vi "Calib_Ref_info.vi"(1 "Input string":string, 2 "Reference Name":string="Instrument to calibrate") -> (0 "Reference instrument":T2={"high limit (10V)"=4.0, "low limit (-10V)"=0.0, "Ch No"=4, "Off ch no"=0, "Calib filename"=path "", "Ref Instrument type"=enum."Enter Value"} {"Off ch no" min=0 max=1; "Ch No" min=0 max=7; "low limit (-10V)" min=-10 max=10 format="%.1f"; "high limit (10V)" min=-10 max=10 format="%.1f"})   [LabVIEW 2010]
uses:
  Calib_setup.ctl
  Controls/Ref_Inst_type.ctl
panel:
  in  "Ref Instrument type":T1=enum."Generic Linear"
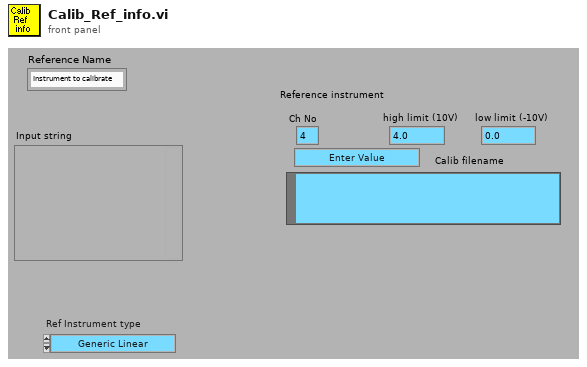
[diagram p1: front panel]
types:
  T1 = typedef "Ref_Inst_type.ctl" = enum16{"Propellor anemometer", "Pressure Transducer", "Raw voltage", "Pitot-static tube", "Preston tube", "Generic Linear", "Generic Polynomial", "Thermocouple", "LDA", "Enter Value", "ADAM Channel"}
  T2 = typedef "Calib_setup.ctl" = cluster{"high limit (10V)":sgl, "low limit (-10V)":sgl, "Ch No":i16, "Off ch no":i8, "Calib filename":path, "Ref Instrument type":T1}
  T3 = cluster{"high limit (10V)":sgl, "low limit (-10V)":sgl, "Ch No":i16, "Off ch no":i8, "Calib filename":path, "Ref Instrument type":enum16{"Propellor anemometer", "Pressure Transducer", "Raw voltage", "Pitot-static tube", "Generic Inst", "Thermocouple", "LDA", "Enter Value", "ADAM Channel"}}
  T4 = enum16{"Propellor anemometer", "Pressure Transducer", "Raw voltage", "Pitot-static tube", "Generic Inst", "Thermocouple", "LDA", "Enter Value", "ADAM Channel"}
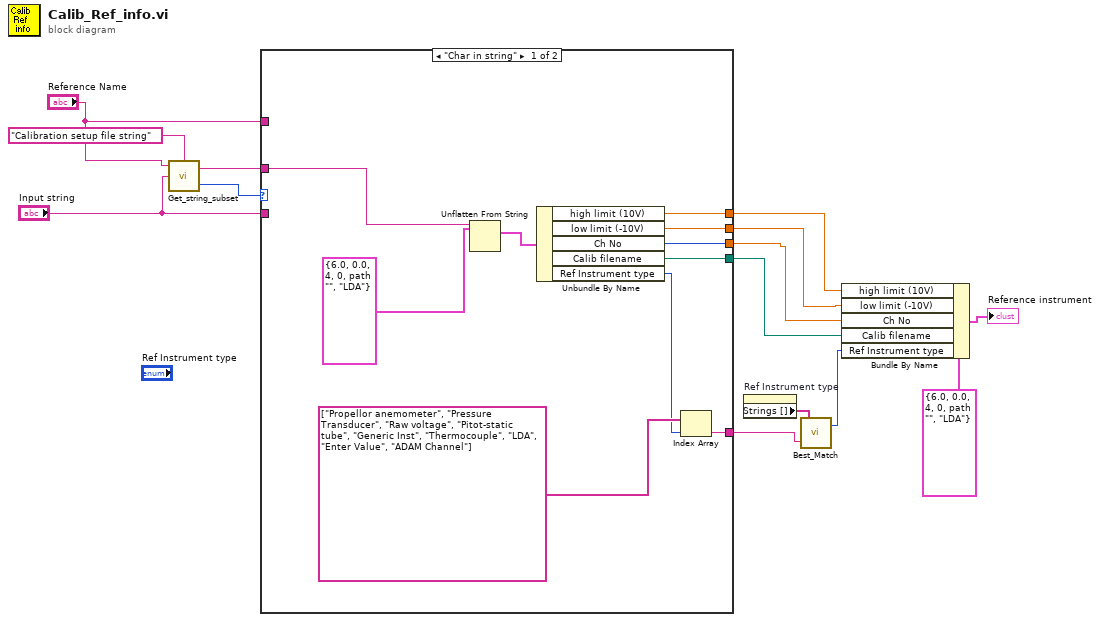
[diagram p0: block diagram]
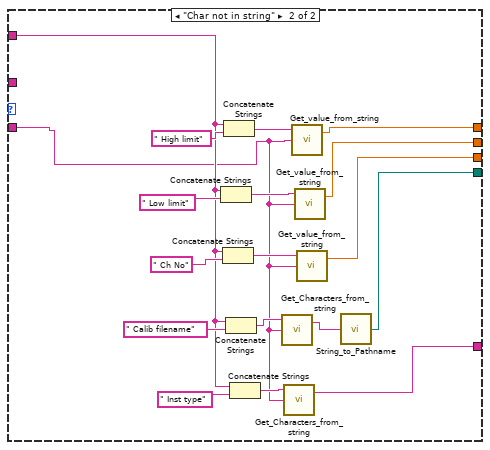
[diagram p2: hidden frame]
diagram:
  n1 = call "Get_string_subset.vi"("String Name"="Calibration setup file string", "String to split"="Input string", "File Label"="Reference Name") -> ("Status"=w13:enum16{"Char in string", "Char not in string"}, "Output string"=w12:string)  [unwired: 1 in]
  n2 = case shown="\"Char in string\"" w13 {
    tunnel: "Input string" -> [_ w30]
    tunnel: w12 -> [w24 _]
    tunnel: "Reference Name" -> [_ w34]
    tunnel: [w19 w25] -> w7
    tunnel: [w18 w26] -> w5
    tunnel: [w17 w27] -> w4
    tunnel: [w16 w28] -> w3
    tunnel: [w15 w29] -> w2
    frame "Char in string" {
      n3 = Unflatten From String(type=T3 {"high limit (10V)"=6.0, "low limit (-10V)"=0.0, "Ch No"=4, "Off ch no"=0, "Calib filename"=path "", "Ref Instrument type"=enum."LDA"} ("Ref vel for angle calib"), binary string=w24) -> (value=w22:T3)  [unwired: 1 in, 4 out]
      n4 = Unbundle By Name(w22) -> ("high limit (10V)"=w15:sgl, "low limit (-10V)"=w16:sgl, "Ch No"=w17:i16, "Calib filename"=w18:path, "Ref Instrument type"=w20:T4)
      n5 = Index Array(array=string[] ["Propellor anemometer", "Pressure Transducer", "Raw voltage", "Pitot-static tube", "Generic Inst", "Thermocouple", "LDA", "Enter Value", "ADAM Channel"] ("Strings []"), index=w20) -> (element=w19:string)
    }
    frame "Char not in string" {
      n6 = Concatenate Strings(w34, " Low limit") -> (w37:string)
      n7 = Concatenate Strings(w34, " Ch No") -> (w38:string)
      n8 = Concatenate Strings(w34, " High limit") -> (w39:string)
      n9 = Concatenate Strings(w34, " Calib filename") -> (w33:string)
      n10 = Concatenate Strings(w34, " Inst type") -> (w31:string)
      n11 = call "Get_Characters_from_string.vi"("Input string"=w30, "Variable name"=w33) -> ("Value"=w32:string)  [unwired: 1 in, 1 out]
      n12 = call "Get_Characters_from_string.vi"("Input string"=w30, "Variable name"=w31) -> ("Value"=w25:string)  [unwired: 1 in, 1 out]
      n13 = call "Get_value_from_string.vi"("Input string"=w30, "Variable name"=w39) -> ("Value"=w29:dbl)  [unwired: 1 in, 1 out]
      n14 = call "Get_value_from_string.vi"("Input string"=w30, "Variable name"=w37) -> ("Value"=w28:dbl)  [unwired: 1 in, 1 out]
      n15 = call "Get_value_from_string.vi"("Input string"=w30, "Variable name"=w38) -> ("Value"=w27:dbl)  [unwired: 1 in, 1 out]
      n16 = call "String_to_Pathname.vi"("Input String"=w32) -> ("path"=w26:path)
    }
  }
  n17 = property on="Ref Instrument type" class="Enum (strict)"() -> ("Strings []"=w8:string[])  [unwired: 2 in, 2 out]
  n18 = call "Best_Match.vi"("Input String"=w7, "String Options"=w8) -> ("index of element"=w6:i32)  [unwired: 1 out]
  n19 = Bundle By Name(cluster=T2 {"high limit (10V)"=6.0, "low limit (-10V)"=0.0, "Ch No"=4, "Off ch no"=0, "Calib filename"=path "", "Ref Instrument type"=enum."LDA"} ("Reference instrument"), "high limit (10V)"=w2, "low limit (-10V)"=w3, "Ch No"=w4, "Calib filename"=w5, "Ref Instrument type"=w6) -> (→"Reference instrument":T2)
